vi "Thermometer Reading with Write to text file.vi"() -> ()   [LabVIEW 2020]
panel:
  out "Waveform Chart":dbl(graph)
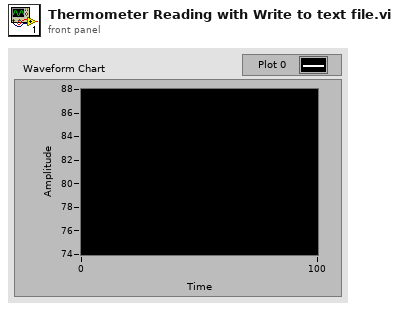
[diagram p1: front panel]
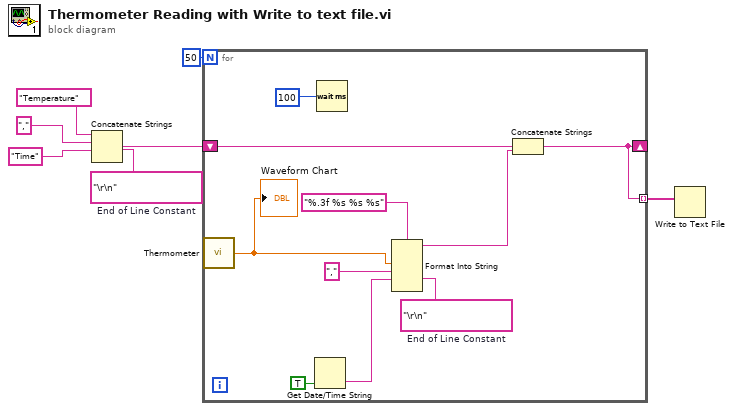
[diagram p0: block diagram]
diagram:
  w3 = "\r\n"  # End of Line Constant
  n1 = Concatenate Strings "Concatenate Strings"("Temperature" ("string"), "," ("string"), "Time" ("string"), w3) -> (w2:string)
  n2 = for {
    N: 50 -> [_]
    shift-right: [w8] -> _
    shift-left: w2 -> [w11]
    tunnel: [w8] -> w1 mode=indexing
    w13 = "\r\n"  # End of Line Constant
    n3 = call "Thermometer.vi"() -> ("Temperature (deg F)"=w9:dbl)  [unwired: 1 in]
    "Waveform Chart" <- w9
    n4 = Get Date/Time String(want seconds? (F)=TRUE) -> (time string=w15:string)  [unwired: 2 in, 1 out]
    n5 = Wait (ms)(milliseconds to wait=u32 100 ("millisecond timer value")) -> ()  [unwired: 1 out]
    n6 = Format Into String "Format Into String"(format string="%.3f %s %s %s", w9, "," ("input 2"), w15, w13) -> (resulting string=w12:string)  [unwired: 2 in, 1 out]
    n7 = Concatenate Strings "Concatenate Strings"(w11, w12) -> (w8:string)
  }
  n8 = Write to Text File(text=w1) -> ()  [unwired: 3 in, 3 out]
